vi "test Data Types.vi"(8 "error in (no error)":errorcluster, 11 "TestCase in":refnum<class "BNR.lvclass">) -> (0 "error out":errorcluster, 3 "TestCase out":refnum<class "BNR.lvclass">)   [LabVIEW 2027, in "BNR.lvclass"]
uses:
  BNR.lvclass
  ea4660e2-e94a-4730-92e4-4a979d9ba497.vi
  dd848d0f-3c36-47ac-a1a5-bdec4e557583.vi
  8853a246-4140-4473-a418-672ac39e676d.vi
  70a56a29-7605-4fb7-a3c2-9569d1e6a598.vi
  8bc1e205-e619-4779-98f3-d88ede699e43.vi
  0ab31b35-db84-45ff-bc08-0ce488ab4d39.vi
  d9da05b8-8c4b-432a-812e-18e8cf1e7732.vi
  e875d667-e5ee-45ee-93e8-1ede48a590f4.vi
  c99423fd-604f-478d-bbad-01e32088edde.vi
  7e27276a-05e4-4bcc-bc7a-cb86725880cf.vi
  e44283f0-00c1-482d-9767-faa7a6297267.vi
  679bdd48-21e9-4857-8799-eae4867f671a.vi
  93659853-5df4-479f-b147-bcd42bc4e5d6.vi
  093b0240-a2ce-4c94-962c-09d44baff142.vi
  19c52a08-f85b-461a-baf2-65c061ff472d.vi
  0aadc548-88a3-48b5-8e87-c47f67ceed28.vi
  60511d20-a68c-4a95-a779-01fd0b81eb24.vi
  ea4660e2-e94a-4730-92e4-4a979d9ba497.vi/9377bb8f-44b5-4a8f-87f1-966fd5a9edcc.vi
  ea4660e2-e94a-4730-92e4-4a979d9ba497.vi/e95d9d1f-307c-44d6-9f26-c3f519a4990d.vi
  ea4660e2-e94a-4730-92e4-4a979d9ba497.vi/0c23f515-4369-4514-bc3d-4444e6b437b2.vi
  dd848d0f-3c36-47ac-a1a5-bdec4e557583.vi/9377bb8f-44b5-4a8f-87f1-966fd5a9edcc.vi
  dd848d0f-3c36-47ac-a1a5-bdec4e557583.vi/e95d9d1f-307c-44d6-9f26-c3f519a4990d.vi
  dd848d0f-3c36-47ac-a1a5-bdec4e557583.vi/0c23f515-4369-4514-bc3d-4444e6b437b2.vi
  8853a246-4140-4473-a418-672ac39e676d.vi/16a2565b-3c16-407b-a626-9da2a3da432e.vi
  70a56a29-7605-4fb7-a3c2-9569d1e6a598.vi/9377bb8f-44b5-4a8f-87f1-966fd5a9edcc.vi
  70a56a29-7605-4fb7-a3c2-9569d1e6a598.vi/e95d9d1f-307c-44d6-9f26-c3f519a4990d.vi
  70a56a29-7605-4fb7-a3c2-9569d1e6a598.vi/0c23f515-4369-4514-bc3d-4444e6b437b2.vi
  8bc1e205-e619-4779-98f3-d88ede699e43.vi/16a2565b-3c16-407b-a626-9da2a3da432e.vi
  0ab31b35-db84-45ff-bc08-0ce488ab4d39.vi/9377bb8f-44b5-4a8f-87f1-966fd5a9edcc.vi
  0ab31b35-db84-45ff-bc08-0ce488ab4d39.vi/e95d9d1f-307c-44d6-9f26-c3f519a4990d.vi
  0ab31b35-db84-45ff-bc08-0ce488ab4d39.vi/0c23f515-4369-4514-bc3d-4444e6b437b2.vi
  d9da05b8-8c4b-432a-812e-18e8cf1e7732.vi/16a2565b-3c16-407b-a626-9da2a3da432e.vi
  e875d667-e5ee-45ee-93e8-1ede48a590f4.vi/9377bb8f-44b5-4a8f-87f1-966fd5a9edcc.vi
  e875d667-e5ee-45ee-93e8-1ede48a590f4.vi/e95d9d1f-307c-44d6-9f26-c3f519a4990d.vi
  e875d667-e5ee-45ee-93e8-1ede48a590f4.vi/0c23f515-4369-4514-bc3d-4444e6b437b2.vi
  c99423fd-604f-478d-bbad-01e32088edde.vi/16a2565b-3c16-407b-a626-9da2a3da432e.vi
  7e27276a-05e4-4bcc-bc7a-cb86725880cf.vi/9377bb8f-44b5-4a8f-87f1-966fd5a9edcc.vi
  7e27276a-05e4-4bcc-bc7a-cb86725880cf.vi/e95d9d1f-307c-44d6-9f26-c3f519a4990d.vi
  7e27276a-05e4-4bcc-bc7a-cb86725880cf.vi/0c23f515-4369-4514-bc3d-4444e6b437b2.vi
  e44283f0-00c1-482d-9767-faa7a6297267.vi/16a2565b-3c16-407b-a626-9da2a3da432e.vi
  679bdd48-21e9-4857-8799-eae4867f671a.vi/9377bb8f-44b5-4a8f-87f1-966fd5a9edcc.vi
  679bdd48-21e9-4857-8799-eae4867f671a.vi/e95d9d1f-307c-44d6-9f26-c3f519a4990d.vi
  679bdd48-21e9-4857-8799-eae4867f671a.vi/0c23f515-4369-4514-bc3d-4444e6b437b2.vi
  93659853-5df4-479f-b147-bcd42bc4e5d6.vi/16a2565b-3c16-407b-a626-9da2a3da432e.vi
  093b0240-a2ce-4c94-962c-09d44baff142.vi/9377bb8f-44b5-4a8f-87f1-966fd5a9edcc.vi
  093b0240-a2ce-4c94-962c-09d44baff142.vi/e95d9d1f-307c-44d6-9f26-c3f519a4990d.vi
  093b0240-a2ce-4c94-962c-09d44baff142.vi/0c23f515-4369-4514-bc3d-4444e6b437b2.vi
  19c52a08-f85b-461a-baf2-65c061ff472d.vi/16a2565b-3c16-407b-a626-9da2a3da432e.vi
  0aadc548-88a3-48b5-8e87-c47f67ceed28.vi/9377bb8f-44b5-4a8f-87f1-966fd5a9edcc.vi
  0aadc548-88a3-48b5-8e87-c47f67ceed28.vi/e95d9d1f-307c-44d6-9f26-c3f519a4990d.vi
  0aadc548-88a3-48b5-8e87-c47f67ceed28.vi/0c23f515-4369-4514-bc3d-4444e6b437b2.vi
  60511d20-a68c-4a95-a779-01fd0b81eb24.vi/16a2565b-3c16-407b-a626-9da2a3da432e.vi
  C:/Program Files/National Instruments/LabVIEW 2027/vi.lib/addons/_JKI Toolkits/VI Tester/TestCase.llb/TestCase.lvclass
  <vilib>/addons/_JKI Toolkits/VI Tester/TestCase.llb/TestCase.lvclass
panel:
  out "BCD encoded value":bool[](array[boolean])
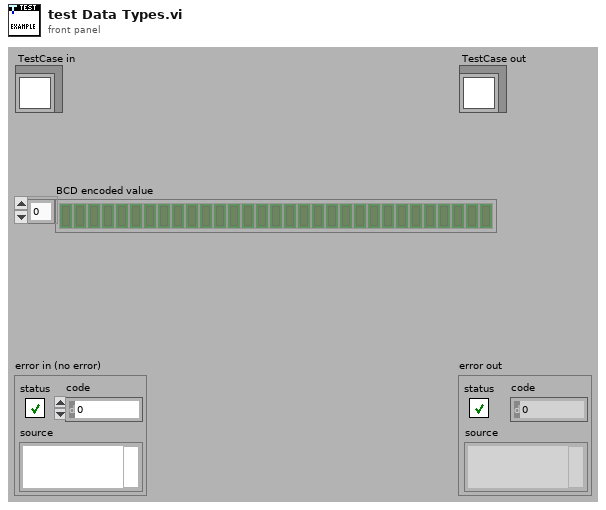
[diagram p1: front panel]
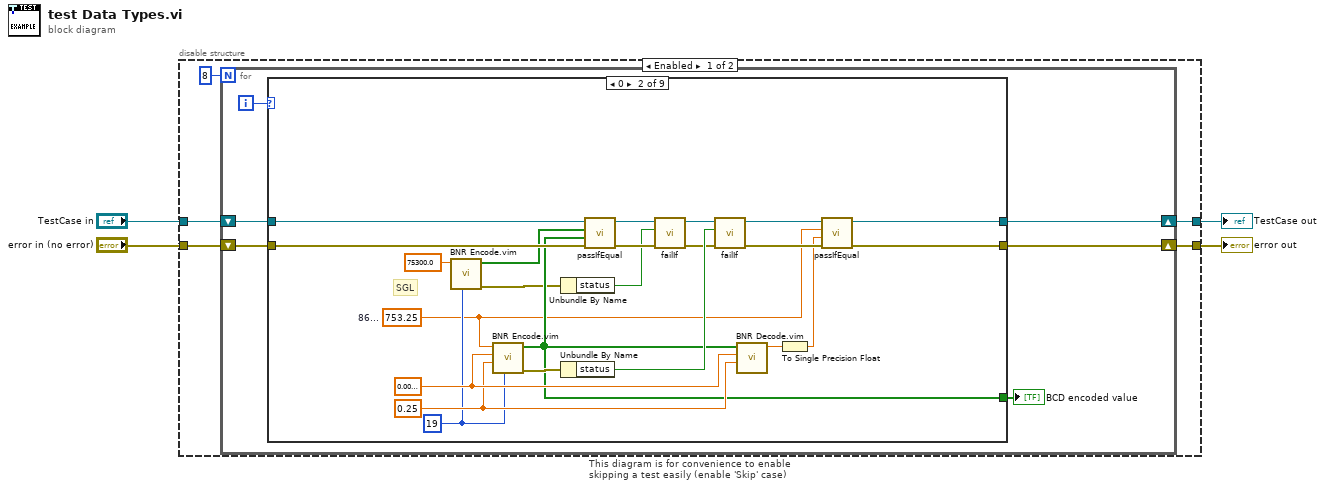
[diagram p0: block diagram]
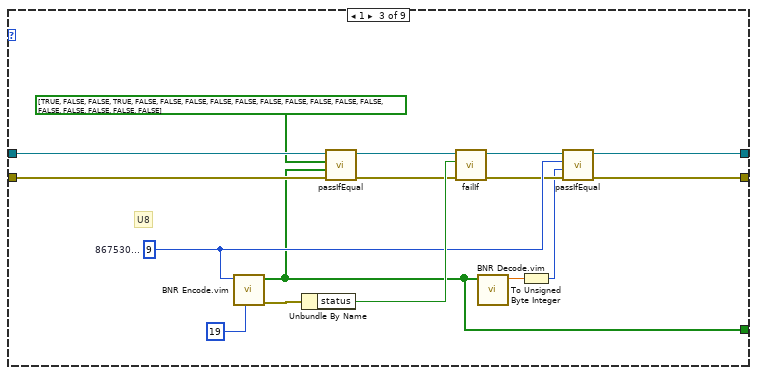
[diagram p3: hidden frame]
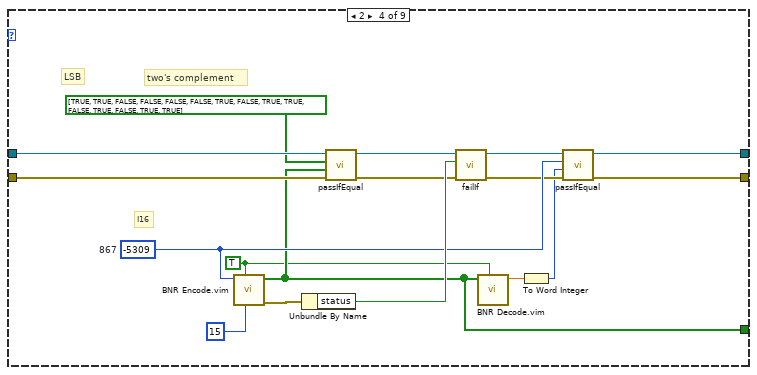
[diagram p4: hidden frame]
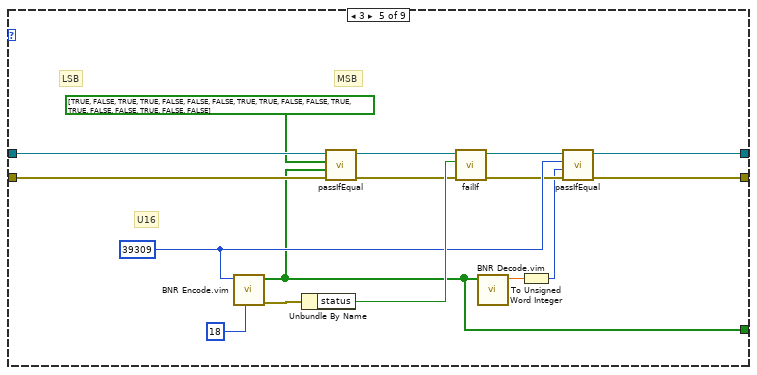
[diagram p5: hidden frame]
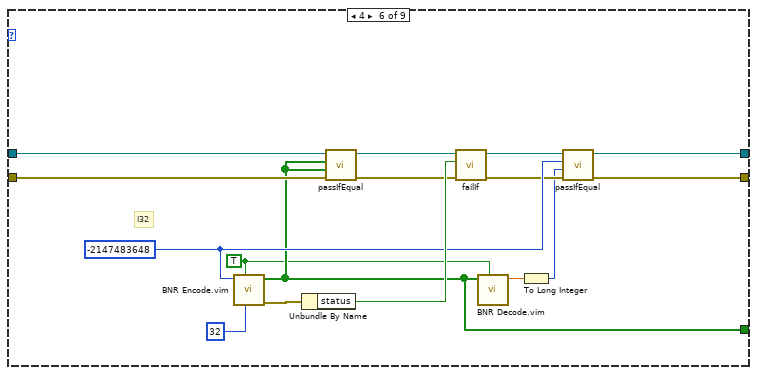
[diagram p6: hidden frame]
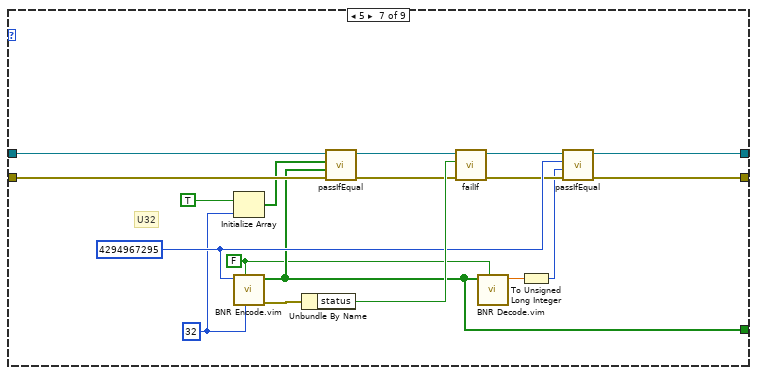
[diagram p7: hidden frame]
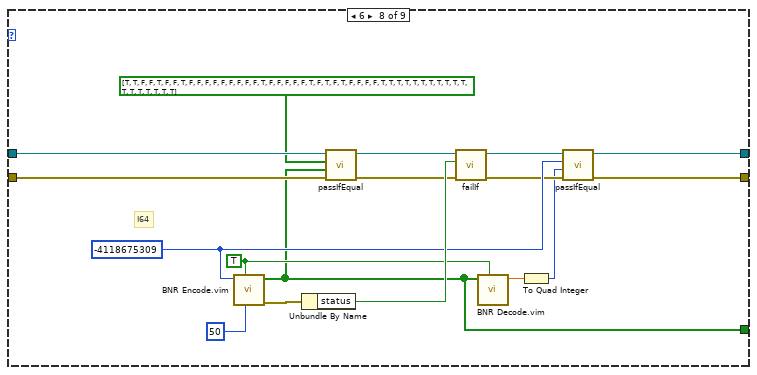
[diagram p8: hidden frame]
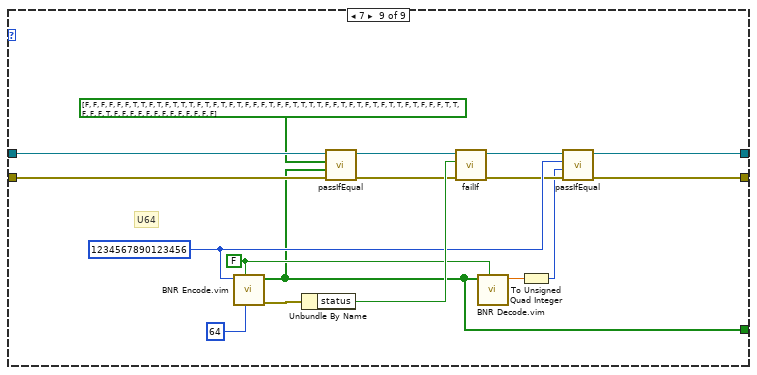
[diagram p9: hidden frame]
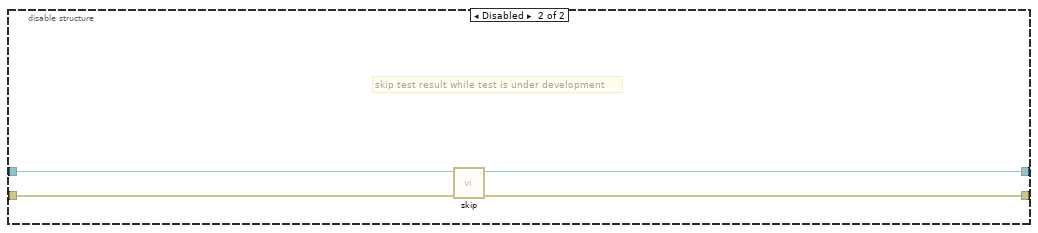
[diagram p10: hidden frame]
diagram:
  n1 = disable-structure "This diagram is for convenience to enable skipping a test easily (enable 'Skip' case)" shown="Enabled" {
    disable-tunnel: "TestCase in" -> [w9 w161]
    disable-tunnel: [w6 w159] -> w3
    disable-tunnel: [w7 w160] -> w1
    disable-tunnel: "error in (no error)" -> [w8 w158]
    frame Enabled {
      n2 = for {
        N: 8 -> [_]
        shift-right: [w12] -> w6
        shift-left: w9 -> [w15]
        shift-right: [w13] -> w7
        shift-left: w8 -> [w14]
        i -> [w11]
        n3 = case shown="0" w11 {
          tunnel: w15 -> [w17 w39 w54 w71 w87 w103 w122 w138 w155]
          tunnel: w14 -> [w16 w38 w53 w70 w86 w102 w121 w137 w154]
          tunnel: [w16 w31 w44 w61 w77 w94 w113 w129 w146] -> w13
          tunnel: [w17 w30 w43 w60 w76 w93 w112 w128 w145] -> w12
          tunnel: [_ w29 w41 w58 w74 w91 w110 w124 w141] -> w10
          frame Default {
          }
          frame 0 {
            w34 = sgl 0.25 ("scale multiplier")
            w35 = sgl 0.01 ("scale multiplier")
            w28 = 19 ("data size (bits)")
            w25 = sgl 753.25  # 86...
            # "SGL"
            n4 = call "BNR Encode.vim"("data size (bits)"=w28, "value"=sgl 75300.0) -> ("error out"=w23:errorcluster, "BNR encoded value"=w26:bool[])  [unwired: 8 in]
            n5 = call "BNR Encode.vim"("data size (bits)"=w28, "scale offset"=w34, "scale multiplier"=w35, "value"=w25) -> ("error out"=w37:errorcluster, "BNR encoded value"=w29:bool[])  [unwired: 6 in]
            n6 = Unbundle By Name(w23) -> ("status"=w18:bool)
            n7 = Unbundle By Name(w37) -> ("status"=w36:bool)
            n8 = call-dynamic "passIfEqual.vi"("error in (no error)"=w38, "y"=w29, "x"=w26, "TestCase in"=w39) -> ("error out"=w21:errorcluster, "TestCase out"=w22:refnum<class "BNR.lvclass">)  [unwired: 6 in]
            n9 = call-dynamic "failIf.vi"("error in (no error)"=w21, "fail"=w18, "TestCase in"=w22) -> ("error out"=w19:errorcluster, "TestCase out"=w20:refnum<class "BNR.lvclass">)  [unwired: 7 in]
            n10 = call-dynamic "failIf.vi"("error in (no error)"=w19, "fail"=w36, "TestCase in"=w20) -> ("error out"=w32:errorcluster, "TestCase out"=w33:refnum<class "BNR.lvclass">)  [unwired: 7 in]
            n11 = call "BNR Decode.vim"("scale offset"=w34, "scale multiplier"=w35, "BNR encoded value"=w29) -> ("value"=w40:dbl)  [unwired: 8 in]
            n12 = To Single Precision Float(number=w40) -> (single precision float=w24:sgl)
            n13 = call-dynamic "passIfEqual.vi"("error in (no error)"=w32, "y"=w24, "x"=w25, "TestCase in"=w33) -> ("error out"=w31:errorcluster, "TestCase out"=w30:refnum<class "BNR.lvclass">)  [unwired: 6 in]
          }
          frame 1 {
            w49 = u8 9  # 867530...
            # "U8"
            n14 = call "BNR Encode.vim"("data size (bits)"=19, "value"=w49) -> ("error out"=w51:errorcluster, "BNR encoded value"=w41:bool[])  [unwired: 8 in]
            n15 = Unbundle By Name(w51) -> ("status"=w50:bool)
            n16 = call-dynamic "passIfEqual.vi"("error in (no error)"=w53, "y"=w41, "x"=bool[] [TRUE, FALSE, FALSE, TRUE, FALSE, FALSE, FALSE, FALSE, FALSE, FALSE, FALSE, FALSE, FALSE, FALSE, FALSE, FALSE, FALSE, FALSE, FALSE] ("BCD encoded value"), "TestCase in"=w54) -> ("error out"=w47:errorcluster, "TestCase out"=w48:refnum<class "BNR.lvclass">)  [unwired: 6 in]
            n17 = call-dynamic "failIf.vi"("error in (no error)"=w47, "fail"=w50, "TestCase in"=w48) -> ("error out"=w45:errorcluster, "TestCase out"=w46:refnum<class "BNR.lvclass">)  [unwired: 7 in]
            n18 = call "BNR Decode.vim"("BNR encoded value"=w41) -> ("value"=w55:dbl)  [unwired: 10 in]
            n19 = To Unsigned Byte Integer(number=w55) -> (unsigned 8bit integer=w42:u8)
            n20 = call-dynamic "passIfEqual.vi"("error in (no error)"=w45, "y"=w42, "x"=w49, "TestCase in"=w46) -> ("error out"=w44:errorcluster, "TestCase out"=w43:refnum<class "BNR.lvclass">)  [unwired: 6 in]
          }
          frame 2 {
            w57 = TRUE ("signed")
            w66 = i16 -5309  # 867
            # "two's complement"
            # "LSB"
            # "I16"
            n21 = call "BNR Encode.vim"("data size (bits)"=15, "signed"=w57, "value"=w66) -> ("error out"=w68:errorcluster, "BNR encoded value"=w58:bool[])  [unwired: 7 in]
            n22 = Unbundle By Name(w68) -> ("status"=w67:bool)
            n23 = call-dynamic "passIfEqual.vi"("error in (no error)"=w70, "y"=w58, "x"=bool[] [TRUE, TRUE, FALSE, FALSE, FALSE, FALSE, TRUE, FALSE, TRUE, TRUE, FALSE, TRUE, FALSE, TRUE, TRUE] ("BCD encoded value"), "TestCase in"=w71) -> ("error out"=w64:errorcluster, "TestCase out"=w65:refnum<class "BNR.lvclass">)  [unwired: 6 in]
            n24 = call-dynamic "failIf.vi"("error in (no error)"=w64, "fail"=w67, "TestCase in"=w65) -> ("error out"=w62:errorcluster, "TestCase out"=w63:refnum<class "BNR.lvclass">)  [unwired: 7 in]
            n25 = call "BNR Decode.vim"("signed"=w57, "BNR encoded value"=w58) -> ("value"=w72:dbl)  [unwired: 9 in]
            n26 = To Word Integer(number=w72) -> (16bit integer=w59:i16)
            n27 = call-dynamic "passIfEqual.vi"("error in (no error)"=w62, "y"=w59, "x"=w66, "TestCase in"=w63) -> ("error out"=w61:errorcluster, "TestCase out"=w60:refnum<class "BNR.lvclass">)  [unwired: 6 in]
          }
          frame 3 {
            w82 = u16 39309 ("867...")
            # "U16"
            # "MSB"
            # "LSB"
            n28 = call "BNR Encode.vim"("data size (bits)"=18, "value"=w82) -> ("error out"=w84:errorcluster, "BNR encoded value"=w74:bool[])  [unwired: 8 in]
            n29 = Unbundle By Name(w84) -> ("status"=w83:bool)
            n30 = call-dynamic "passIfEqual.vi"("error in (no error)"=w86, "y"=w74, "x"=bool[] [TRUE, FALSE, TRUE, TRUE, FALSE, FALSE, FALSE, TRUE, TRUE, FALSE, FALSE, TRUE, TRUE, FALSE, FALSE, TRUE, FALSE, FALSE] ("BCD encoded value"), "TestCase in"=w87) -> ("error out"=w80:errorcluster, "TestCase out"=w81:refnum<class "BNR.lvclass">)  [unwired: 6 in]
            n31 = call-dynamic "failIf.vi"("error in (no error)"=w80, "fail"=w83, "TestCase in"=w81) -> ("error out"=w78:errorcluster, "TestCase out"=w79:refnum<class "BNR.lvclass">)  [unwired: 7 in]
            n32 = call "BNR Decode.vim"("BNR encoded value"=w74) -> ("value"=w88:dbl)  [unwired: 10 in]
            n33 = To Unsigned Word Integer(number=w88) -> (unsigned 16bit integer=w75:u16)
            n34 = call-dynamic "passIfEqual.vi"("error in (no error)"=w78, "y"=w75, "x"=w82, "TestCase in"=w79) -> ("error out"=w77:errorcluster, "TestCase out"=w76:refnum<class "BNR.lvclass">)  [unwired: 6 in]
          }
          frame 4 {
            w90 = TRUE ("signed")
            w99 = -2147483648 ("867...")
            # "I32"
            n35 = call "BNR Encode.vim"("data size (bits)"=32, "signed"=w90, "value"=w99) -> ("error out"=w101:errorcluster, "BNR encoded value"=w91:bool[])  [unwired: 7 in]
            n36 = Unbundle By Name(w101) -> ("status"=w100:bool)
            n37 = call-dynamic "passIfEqual.vi"("error in (no error)"=w102, "y"=w91, "x"=w91, "TestCase in"=w103) -> ("error out"=w97:errorcluster, "TestCase out"=w98:refnum<class "BNR.lvclass">)  [unwired: 6 in]
            n38 = call-dynamic "failIf.vi"("error in (no error)"=w97, "fail"=w100, "TestCase in"=w98) -> ("error out"=w95:errorcluster, "TestCase out"=w96:refnum<class "BNR.lvclass">)  [unwired: 7 in]
            n39 = call "BNR Decode.vim"("signed"=w90, "BNR encoded value"=w91) -> ("value"=w104:dbl)  [unwired: 9 in]
            n40 = To Long Integer(number=w104) -> (32bit integer=w92:i32)
            n41 = call-dynamic "passIfEqual.vi"("error in (no error)"=w95, "y"=w92, "x"=w99, "TestCase in"=w96) -> ("error out"=w94:errorcluster, "TestCase out"=w93:refnum<class "BNR.lvclass">)  [unwired: 6 in]
          }
          frame 5 {
            w109 = FALSE ("signed")
            w107 = 32 ("data size (bits)")
            w118 = u32 4294967295 ("867...")
            # "U32"
            n42 = Initialize Array(TRUE ("signed"), w107) -> (w106:bool[])
            n43 = call "BNR Encode.vim"("data size (bits)"=w107, "signed"=w109, "value"=w118) -> ("error out"=w120:errorcluster, "BNR encoded value"=w110:bool[])  [unwired: 7 in]
            n44 = Unbundle By Name(w120) -> ("status"=w119:bool)
            n45 = call-dynamic "passIfEqual.vi"("error in (no error)"=w121, "y"=w110, "x"=w106, "TestCase in"=w122) -> ("error out"=w116:errorcluster, "TestCase out"=w117:refnum<class "BNR.lvclass">)  [unwired: 6 in]
            n46 = call-dynamic "failIf.vi"("error in (no error)"=w116, "fail"=w119, "TestCase in"=w117) -> ("error out"=w114:errorcluster, "TestCase out"=w115:refnum<class "BNR.lvclass">)  [unwired: 7 in]
            n47 = call "BNR Decode.vim"("signed"=w109, "BNR encoded value"=w110) -> ("value"=w123:dbl)  [unwired: 9 in]
            n48 = To Unsigned Long Integer(number=w123) -> (unsigned 32bit integer=w111:u32)
            n49 = call-dynamic "passIfEqual.vi"("error in (no error)"=w114, "y"=w111, "x"=w118, "TestCase in"=w115) -> ("error out"=w113:errorcluster, "TestCase out"=w112:refnum<class "BNR.lvclass">)  [unwired: 6 in]
          }
          frame 6 {
            w126 = TRUE ("signed")
            w134 = i64 -4118675309 ("867...")
            # "I64"
            n50 = call "BNR Encode.vim"("data size (bits)"=50, "signed"=w126, "value"=w134) -> ("error out"=w136:errorcluster, "BNR encoded value"=w124:bool[])  [unwired: 7 in]
            n51 = Unbundle By Name(w136) -> ("status"=w135:bool)
            n52 = call-dynamic "passIfEqual.vi"("error in (no error)"=w137, "y"=w124, "x"=bool[] [TRUE, TRUE, FALSE, FALSE, TRUE, FALSE, FALSE, TRUE, FALSE, FALSE, FALSE, FALSE, FALSE, FALSE, FALSE, FALSE, FALSE, TRUE, FALSE, FALSE, FALSE, FALSE, FALSE, TRUE, FALSE, TRUE, FALSE, TRUE, FALSE, FALSE, FALSE, FALSE, TRUE, TRUE, TRUE, TRUE, TRUE, TRUE, TRUE, TRUE, TRUE, TRUE, TRUE, TRUE, TRUE, TRUE, TRUE, TRUE, TRUE, TRUE] ("BCD encoded value"), "TestCase in"=w138) -> ("error out"=w132:errorcluster, "TestCase out"=w133:refnum<class "BNR.lvclass">)  [unwired: 6 in]
            n53 = call-dynamic "failIf.vi"("error in (no error)"=w132, "fail"=w135, "TestCase in"=w133) -> ("error out"=w130:errorcluster, "TestCase out"=w131:refnum<class "BNR.lvclass">)  [unwired: 7 in]
            n54 = call "BNR Decode.vim"("signed"=w126, "BNR encoded value"=w124) -> ("value"=w139:dbl)  [unwired: 9 in]
            n55 = To Quad Integer(1:w139) -> (0:w127:i64)
            n56 = call-dynamic "passIfEqual.vi"("error in (no error)"=w130, "y"=w127, "x"=w134, "TestCase in"=w131) -> ("error out"=w129:errorcluster, "TestCase out"=w128:refnum<class "BNR.lvclass">)  [unwired: 6 in]
          }
          frame 7 {
            w143 = FALSE ("signed")
            w151 = u64 1234567890123456 ("867...")
            # "U64"
            n57 = call "BNR Encode.vim"("data size (bits)"=64, "signed"=w143, "value"=w151) -> ("error out"=w153:errorcluster, "BNR encoded value"=w141:bool[])  [unwired: 7 in]
            n58 = Unbundle By Name(w153) -> ("status"=w152:bool)
            n59 = call-dynamic "passIfEqual.vi"("error in (no error)"=w154, "y"=w141, "x"=bool[] [FALSE, FALSE, FALSE, FALSE, FALSE, FALSE, TRUE, TRUE, FALSE, TRUE, FALSE, TRUE, TRUE, TRUE, FALSE, TRUE, FALSE, TRUE, FALSE, TRUE, FALSE, FALSE, FALSE, TRUE, FALSE, FALSE, TRUE, TRUE, TRUE, TRUE, FALSE, FALSE, TRUE, FALSE, TRUE, FALSE, TRUE, FALSE, TRUE, TRUE, FALSE, TRUE, FALSE, FALSE, FALSE, TRUE, TRUE, FALSE, FALSE, FALSE, TRUE, FALSE, FALSE, FALSE, FALSE, FALSE, FALSE, FALSE, FALSE, FALSE, FALSE, FALSE, FALSE, FALSE] ("BCD encoded value"), "TestCase in"=w155) -> ("error out"=w149:errorcluster, "TestCase out"=w150:refnum<class "BNR.lvclass">)  [unwired: 6 in]
            n60 = call-dynamic "failIf.vi"("error in (no error)"=w149, "fail"=w152, "TestCase in"=w150) -> ("error out"=w147:errorcluster, "TestCase out"=w148:refnum<class "BNR.lvclass">)  [unwired: 7 in]
            n61 = call "BNR Decode.vim"("signed"=w143, "BNR encoded value"=w141) -> ("value"=w156:dbl)  [unwired: 9 in]
            n62 = To Unsigned Quad Integer(1:w156) -> (0:w144:u64)
            n63 = call-dynamic "passIfEqual.vi"("error in (no error)"=w147, "y"=w144, "x"=w151, "TestCase in"=w148) -> ("error out"=w146:errorcluster, "TestCase out"=w145:refnum<class "BNR.lvclass">)  [unwired: 6 in]
          }
        }
        "BCD encoded value" <- w10
      }
    }
    frame Disabled {
      # "skip test result while test is under development"
      n64 = call <vilib>:"skip.vi"("error in (no error)"=w158, "TestCase in"=w161) -> ("error out"=w160:errorcluster, "TestCase out"=w159:refnum<class "BNR.lvclass">)  [unwired: 8 in]
    }
  }
  "error out" <- w1
  "TestCase out" <- w3
